vi "FTW-Test-Subscriber-ConnectedNoMessages.vi"() -> ()   [LabVIEW 2015]
uses:
  source/actor/Subscriber/FTW-Subscriber.lvclass
  source/actor/Ether/FTW-Ether.lvclass
  source/actor/Publisher/FTW-Publisher.lvclass
panel:
  out "Elapsed Time":dbl format="%<%H:%M:%S%3u>t"
  in  "Number of Subscribers":i32=10
  in  "Wait Time (ms)":u32=1000
  out "Results":T1(array[cluster])
  in  "Addresses":string[](array[string])=["inproc://*", "tcp://127.0.0.1/*"]
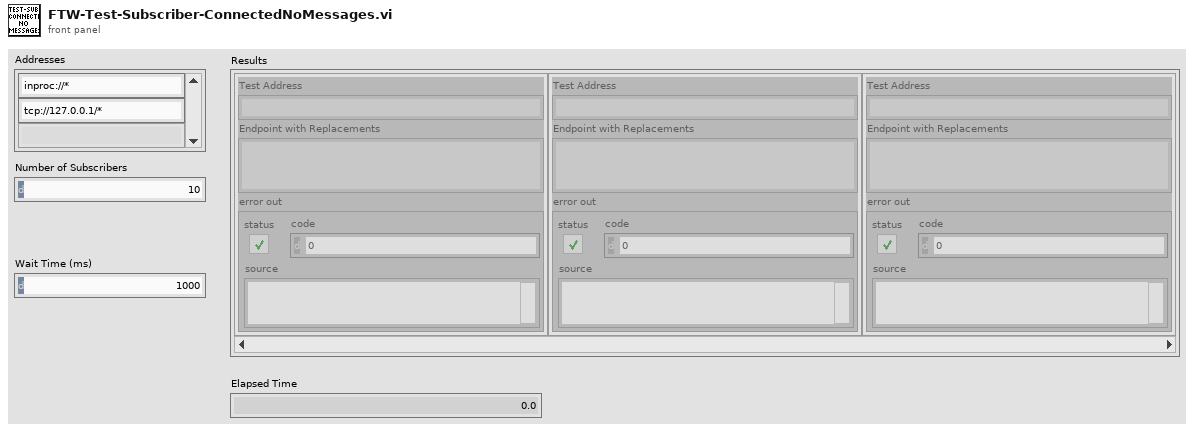
[diagram p1: front panel]
types:
  T1 = cluster{"Test Address":string, "Endpoint with Replacements":string, "error out":errorcluster}[]
  T2 = cluster{"String":string, "Endpoint with Replacements":string, "error IO":errorcluster}
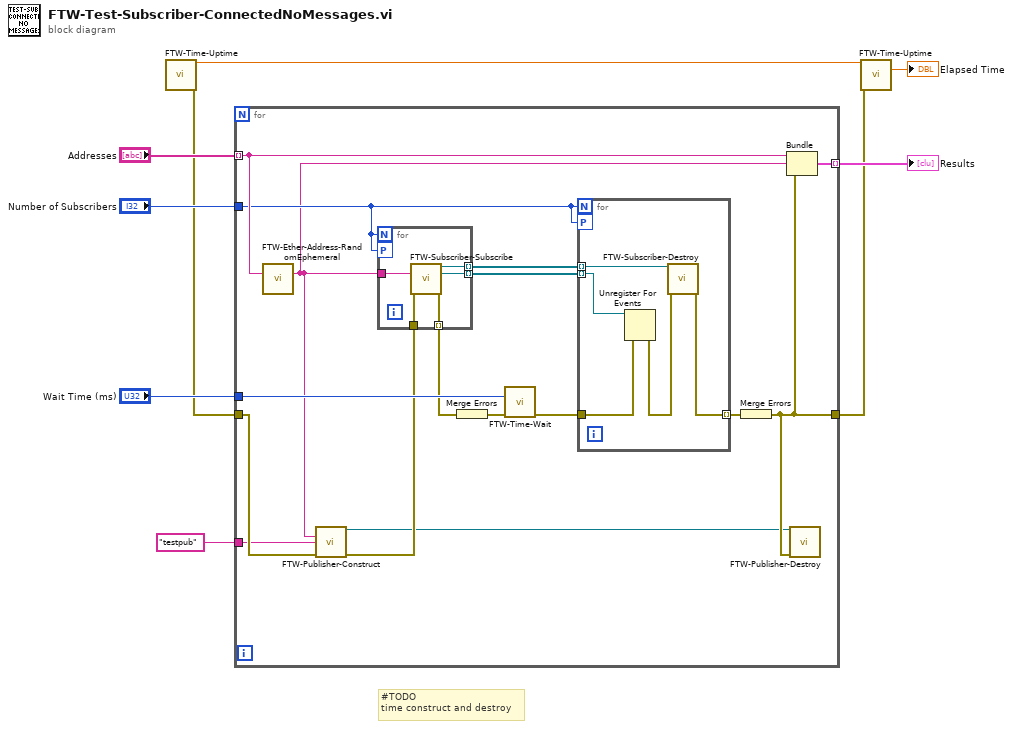
[diagram p0: block diagram]
diagram:
  # "#TODO\ntime construct and destroy"
  n1 = call "FTW-Time-Uptime.vi"() -> ("Current Uptime"=w3:dbl, "error out"=w5:errorcluster)  [unwired: 13 in, 1 out]
  n2 = for {
    tunnel: "Addresses" -> [w25] mode=indexing
    tunnel: [w23] -> w8 mode=indexing
    tunnel: "Wait Time (ms)" -> [w22]
    tunnel: "Number of Subscribers" -> [w16]
    tunnel: w5 -> [w14]
    tunnel: [w11] -> w4
    tunnel: "testpub" ("Identity") -> [w13]
    n3 = call "FTW-Ether-Address-RandomEphemeral.vi"("Endpoint"=w25) -> ("Endpoint with Replacements"=w15:string)  [unwired: 13 in, 1 out]
    n4 = call "FTW-Publisher-Construct.vi"("Address"=w15, "Identity"=w13, "error in"=w14) -> ("FTW-Publisher Out"=w10:refnum<class "FTW-Publisher.lvclass">, "error out"=w12:errorcluster)  [unwired: 10 in, 1 out]
    n5 = for {
      N: w16 -> [_]
      tunnel: w15 -> [w35]
      tunnel: [w34] -> w21 mode=indexing
      tunnel: [w33] -> w19 mode=indexing
      tunnel: [w32] -> w18 mode=indexing
      workers-P: w16 -> [_]
      tunnel: w12 -> [w31]
      n6 = call "FTW-Subscriber-Subscribe.vi"("Addresses"=w35, "error in"=w31) -> ("FTW-Subscription Out"=w32:refnum<class "FTW-Subscriber.lvclass">, "Subscriber Registration"=w33:refnum<event-registration>, "error out"=w34:errorcluster)  [unwired: 11 in]
    }
    n7 = Merge Errors(w21) -> (w17:errorcluster)
    n8 = call "FTW-Time-Wait.vi"("Wait Time (ms)"=w22, "error in"=w17) -> ("error out"=w20:errorcluster)  [unwired: 13 in]
    n9 = for {
      N: w16 -> [_]
      tunnel: [w30] -> w24 mode=indexing
      tunnel: w20 -> [w29]
      tunnel: w19 -> [w27] mode=indexing
      tunnel: w18 -> [w26] mode=indexing
      workers-P: w16 -> [_]
      n10 = Unregister For Events(event registration refnum=w27, error in=w29) -> (error out=w28:errorcluster)
      n11 = call "FTW-Subscriber-Destroy.vi"("FTW-Subscription In"=w26, "error in"=w28) -> ("error out"=w30:errorcluster)  [unwired: 13 in]
    }
    n12 = Merge Errors(w24) -> (w11:errorcluster)
    n13 = Bundle("String"=w25, "Endpoint with Replacements"=w15, "error IO"=w11) -> (w23:T2)  [unwired: 1 in]
    n14 = call "FTW-Publisher-Destroy.vi"("FTW-Publisher In"=w10, "error in"=w11) -> ()  [unwired: 13 in, 1 out]
  }
  "Results" <- w8
  n15 = call "FTW-Time-Uptime.vi"("Previous Uptime"=w3, "error in"=w4) -> ("Elapsed Time"=→"Elapsed Time":dbl)  [unwired: 11 in, 2 out]
